vi "Set Voltage and Current.vi"(0 "Tektronix PA1000 in":refnum<class "Tektronix PA1000.lvclass">, 5 "Card #":u8, 7 "Voltage enum number":u16, 9 "Current enum number":u16, 11 "error in (no error)":errorcluster) -> (4 "Tektronix PA1000 out":refnum<class "Tektronix PA1000.lvclass">, 15 "error out":errorcluster)   [LabVIEW 2013, in "Generic Power Analyzer.lvlib" / "Tektronix PA1000.lvlib" / "Tektronix PA1000.lvclass"]
uses:
  Tektronix PA1000.lvclass
  Generic Power Analyzer/Generic Power Analyzer.lvclass
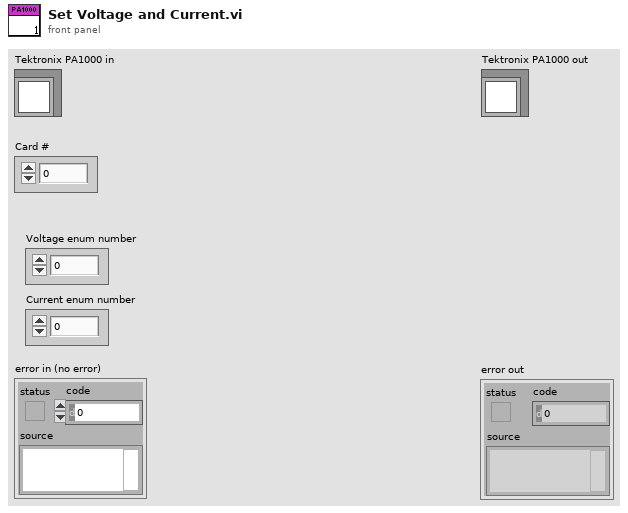
[diagram p1: front panel]
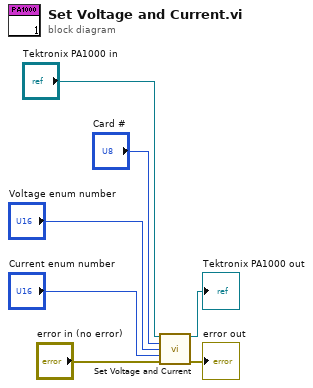
[diagram p0: block diagram]
diagram:
  n1 = call-parent "Set Voltage and Current.vi"("Generic Instrument in"="Tektronix PA1000 in", "Card #"="Card #", "Voltage enum number"="Voltage enum number", "Current enum number"="Current enum number", "error in (no error)"="error in (no error)") -> ("Generic Instrument out"=→"Tektronix PA1000 out":refnum<class "Tektronix PA1000.lvclass">, "error out"=→"error out":errorcluster)  [unwired: 9 in]
